vi "Percorso e nome report.vi"(9 "Default":string[][](array[string]), 10 "Criteri":string[][](array[string]), 11 "DT":string[][](array[string])) -> (1 "path gestionale":path, 2 "path Standard":path, 3 "Nome file":string)   [LabVIEW 2019]
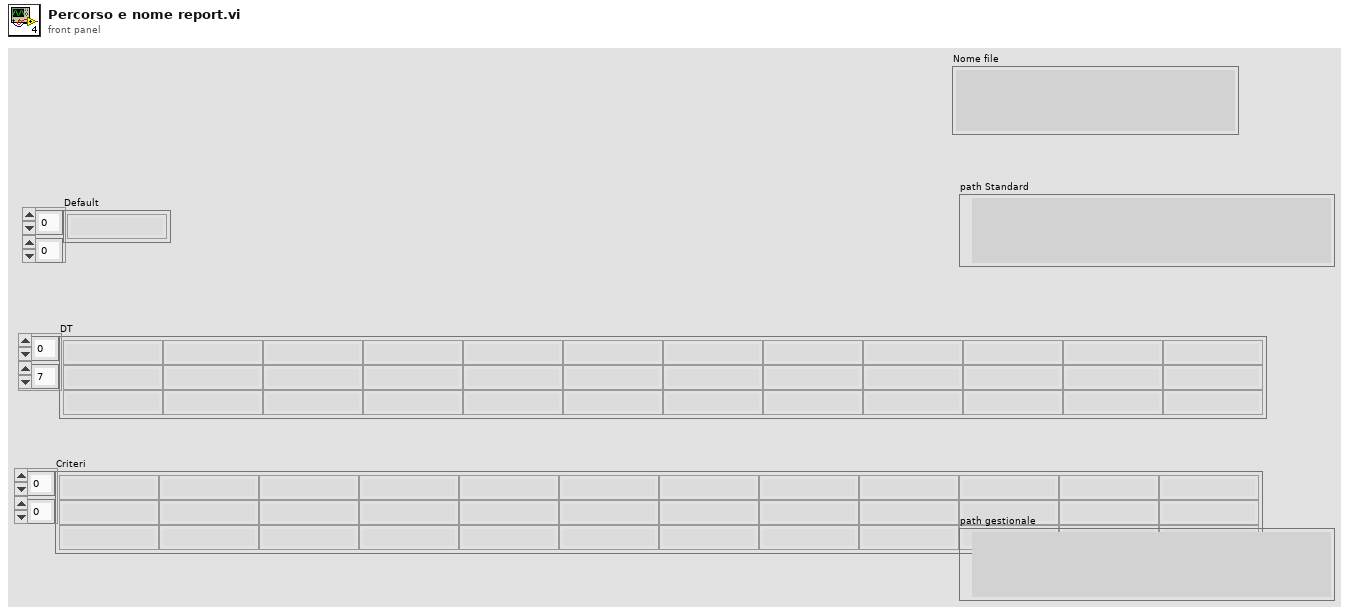
[diagram p1: front panel]
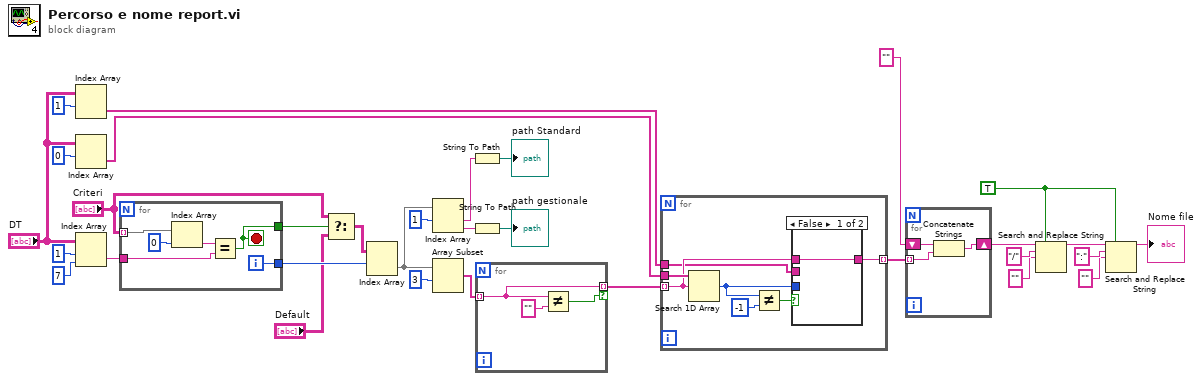
[diagram p0: block diagram]
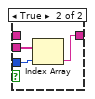
[diagram p2: hidden frame]
diagram:
  w1 = TRUE ("replace all? (F)")
  n1 = Index Array(array="DT", index (row)=1) -> (element=w17:string[])  [unwired: 1 in]
  n2 = Index Array(array="DT", index (row)=0) -> (element=w21:string[])  [unwired: 1 in]
  n3 = Index Array(array="DT", index (row)=1, index (col)=7 ("disabled index (col)")) -> (element=w31:string)
  n4 = for {
    tunnel: "Criteri" -> [w38] mode=indexing
    tunnel: w31 -> [w35]
    tunnel: [w34] -> w26
    tunnel: [w33] -> w29
    i -> [w33]
    stop <- w34 stop-if-true
    n5 = Index Array(array=w38, index=0) -> (element=w36:string)
    n6 = Equal?(x=w36, y=w35) -> (x = y?=w34:bool)
  }
  n7 = Select(t="Criteri", s=w26, f="Default") -> (s? t:f=w23:string[][])
  n8 = Index Array(array=w23, index (row)=w29) -> (element=w12:string[])  [unwired: 1 in]
  n9 = Index Array(array=w12, index #1=1 ("disabled index (col)")) -> (element #1=w22:string, element #2=w10:string)  [unwired: 1 in]
  n10 = Array Subset(array=w12, index=3) -> (w16:string[])  [unwired: 1 in]
  n11 = String To Path(string=w22) -> (path=→"path Standard":path)
  n12 = String To Path(string=w10) -> (path=→"path gestionale":path)
  n13 = for {
    tunnel: w16 -> [w40] mode=indexing
    tunnel: [w40] -> w15 mode=indexing if=w39
    n14 = Not Equal?(x=w40, y="") -> (x != y?=w39:bool)
  }
  n15 = for {
    tunnel: w21 -> [w48]
    tunnel: w15 -> [w43] mode=indexing
    tunnel: [w44] -> w14 mode=indexing
    tunnel: w17 -> [w42]
    n16 = Search 1D Array(1D array=w48, element=w43) -> (index of element=w47:i32)  [unwired: 1 in]
    n17 = Not Equal?(x=w47, y=-1) -> (x != y?=w45:bool)
    n18 = case shown="False" w45 {
      tunnel: w47 -> [_ w50]
      tunnel: [w49 w52] -> w44
      tunnel: w43 -> [w49 _]
      tunnel: w42 -> [_ w51]
      frame False {
      }
      frame True {
        n19 = Index Array(array=w51, index=w50) -> (element=w52:string)
      }
    }
  }
  n20 = for {
    tunnel: w14 -> [w53] mode=indexing
    shift-right: [w54] -> w8
    shift-left: "" -> [w55]
    n21 = Concatenate Strings(w55, w53) -> (w54:string)
  }
  n22 = Search and Replace String(replace all?=w1, input string=w8, search string="/", replace string="" ("replace string (\"\")")) -> (result string=w5:string)  [unwired: 4 in, 3 out]
  n23 = Search and Replace String(replace all?=w1, input string=w5, search string=":", replace string="" ("replace string (\"\")")) -> (result string=→"Nome file":string)  [unwired: 4 in, 3 out]
